vi "_unloadStage.vi"(8 "error in (no error)":errorcluster, 11 "ESP301_via_TCPIP in":refnum<class "ESP301_via_TCPIP.lvclass">) -> (0 "error out":errorcluster, 3 "ESP301_via_TCPIP out":refnum<class "ESP301_via_TCPIP.lvclass">)   [LabVIEW 2018, in "ESP301_via_TCPIP.lvclass"]
uses:
  ESP301_via_TCPIP.lvclass
  _delayStageBase/_delayStageBase.lvclass
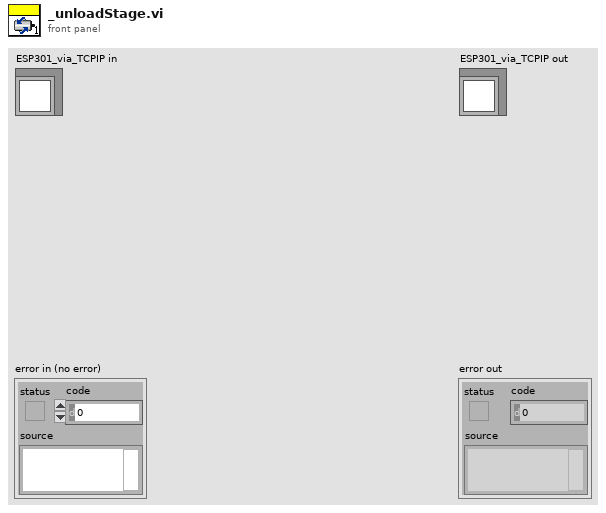
[diagram p1: front panel]
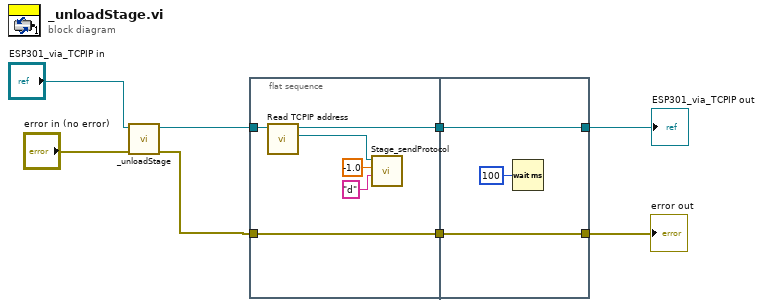
[diagram p0: block diagram]
diagram:
  n1 = call-parent "_unloadStage.vi"("error in (no error)"="error in (no error)", "_delayStageBase in"="ESP301_via_TCPIP in") -> ("error out"=w3:errorcluster, "_delayStageBase out"=w6:refnum<class "ESP301_via_TCPIP.lvclass">)  [unwired: 8 in]
  n2 = flat-sequence {
    tunnel: w6 -> [w13]
    tunnel: [w12] -> w4
    tunnel: w3 -> [w9]
    tunnel: [w9] -> w2
    tunnel: [w17] -> w5
    tunnel: w4 -> [w17]
    tunnel: w2 -> [w16]
    tunnel: [w16] -> w1
    frame #0 {
      n3 = call-dynamic "Read TCPIP address.vi"("ESP301_via_TCPIP in"=w13) -> ("TCPIP address"=w14:refnum<k5>, "ESP301_via_TCPIP out"=w12:refnum<class "ESP301_via_TCPIP.lvclass">)  [unwired: 8 in, 1 out]
      n4 = call "Stage_sendProtocol.vi"("command"="d", "GoTo position"=-1.0, "TCP Network Connection in"=w14) -> ()  [unwired: 7 in, 2 out]
    }
    frame #1 {
      n5 = Wait (ms)(milliseconds to wait=u32 100) -> ()  [unwired: 1 out]
    }
  }
  "error out" <- w1
  "ESP301_via_TCPIP out" <- w5
